vi "combined arm safety.vi"(1 "Input":dbl) -> (0 "Safe Output":dbl)   [LabVIEW 2013]
panel:
  in  "Min Rate":dbl format="%#_13g"
  in  "Max Rate":dbl=50.0 format="%#_13g"
  in  "Forward Limit":dbl format="%#_13g"
  in  "Reverse Limit":dbl format="%#_13g"
  in  "Cutoff Rate":dbl=0.8 format="%#_13g"
  # "Things needing Tuning"
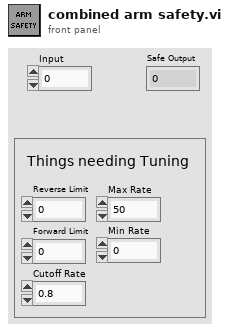
[diagram p1: front panel]
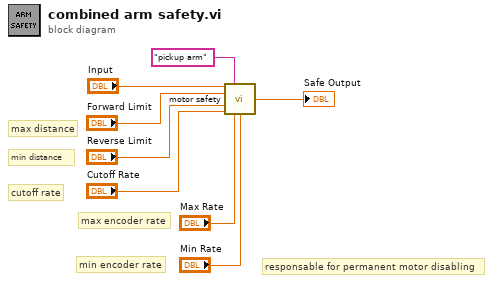
[diagram p0: block diagram]
diagram:
  # "responsable for permanent motor disabling"
  # "min encoder rate"
  # "max encoder rate"
  # "cutoff rate"
  # "min distance"
  # "max distance"
  n1 = call "motor safety.vi"("Desired Rate"="Input", "Encoder Refnum"="pickup arm", "Forward Limit"="Forward Limit", "Reverse Limit"="Reverse Limit", "Cutoff Rate"="Cutoff Rate", "Max Rate"="Max Rate", "Min Rate"="Min Rate") -> ("Rate Output"=→"Safe Output":dbl)  [unwired: 8 in]
